vi "Test ReInit Negative Responce and ReInit.vi"(7 "Sequence Context In":refnum<k7>, 8 "error in":errorcluster, 9 "Test Mode":u16, 10 "LV PPS Config":T1={"VISA Resource"="", "Voltage Level (0.0 V)"=12.0, "CURRent Limit (0.0 A)"=6.0, "OVP LEVEL (0V)"=15.0, "Enable OVP (T: Enable)"=FALSE, "OCP LEVEL (0A)"=8.0, "Enable OCP (T: Enable)"=TRUE, "Value Out"="", "Value In"="", "Actual Voltage Level (V)"=-0.11, "Actual Current Limit (A)"=0.0, "Select Instrument"="", "Enable Output"=TRUE, "PPS Operation"=enum."Configure", "Type"=0} {"Type" items=["Voltage", "Current"]; "Actual Current Limit (A)" format="%.2f"; "Actual Voltage Level (V)" format="%.2f"; "OCP LEVEL (0A)" format="%.2f"; "OVP LEVEL (0V)" format="%.2f"; "Voltage Level (0.0 V)" format="%.2f"}, 11 "HV PPS Config":T1={"VISA Resource"="", "Voltage Level (0.0 V)"=48.0, "CURRent Limit (0.0 A)"=150.0, "OVP LEVEL (0V)"=55.0, "Enable OVP (T: Enable)"=FALSE, "OCP LEVEL (0A)"=160.0, "Enable OCP (T: Enable)"=TRUE, "Value Out"="", "Value In"="", "Actual Voltage Level (V)"=-0.11, "Actual Current Limit (A)"=0.0, "Select Instrument"="", "Enable Output"=TRUE, "PPS Operation"=enum."Configure", "Type"=0} {"Type" items=["Voltage", "Current"]; "Actual Current Limit (A)" format="%.2f"; "Actual Voltage Level (V)" format="%.2f"; "OCP LEVEL (0A)" format="%.2f"; "OVP LEVEL (0V)" format="%.2f"; "Voltage Level (0.0 V)" format="%.2f"}) -> (0 "error out":errorcluster, 2 "Response Code":u8[](array[numeric]), 3 "Positive Responce":bool)   [LabVIEW 2023, in "HardwareAbstractionLayer_LVOOP.lvlib" / "Wait Monitor.lvclass"]
uses:
  Wait Monitor.lvclass
  PowerSupply/Teststand/Control/PPS StepType Control.ctl
  Teststand Steptypes/CAN/STP/Steptypes/Control/STP Data.ctl
  CAN/CAN Application Protocols/STP Protocol_class/Ctrls/STP CMD.ctl
  Teststand Steptypes/DAQ/Relay Output/Control/Relay Output.ctl
  c292acb4-9eb8-428b-88b9-75ff1cad1871.vi
  57b82cc3-dd7c-4d3a-8ba9-81b38abffcad.vi
  725d82db-e125-4af1-8c31-2eddca650097.vi
  e56fdc52-0104-40be-a5d4-315e7d7fad48.vi
  ae1cdcb4-d38d-44ac-ba66-047396e49866.vi
  74cc3969-7d3f-4b2d-8c71-1ae829f8c662.vi
  02209c7f-5af8-4368-83f9-8143192c00df.vi
  Teststand/Teststand.lvclass
  CAN/CAN Application Protocols/STP Protocol_class/STP Protocol.lvclass
  Teststand Steptypes/LTT_TeststandSteptypes.lvlib
  PowerSupply/PowerSupply.lvclass
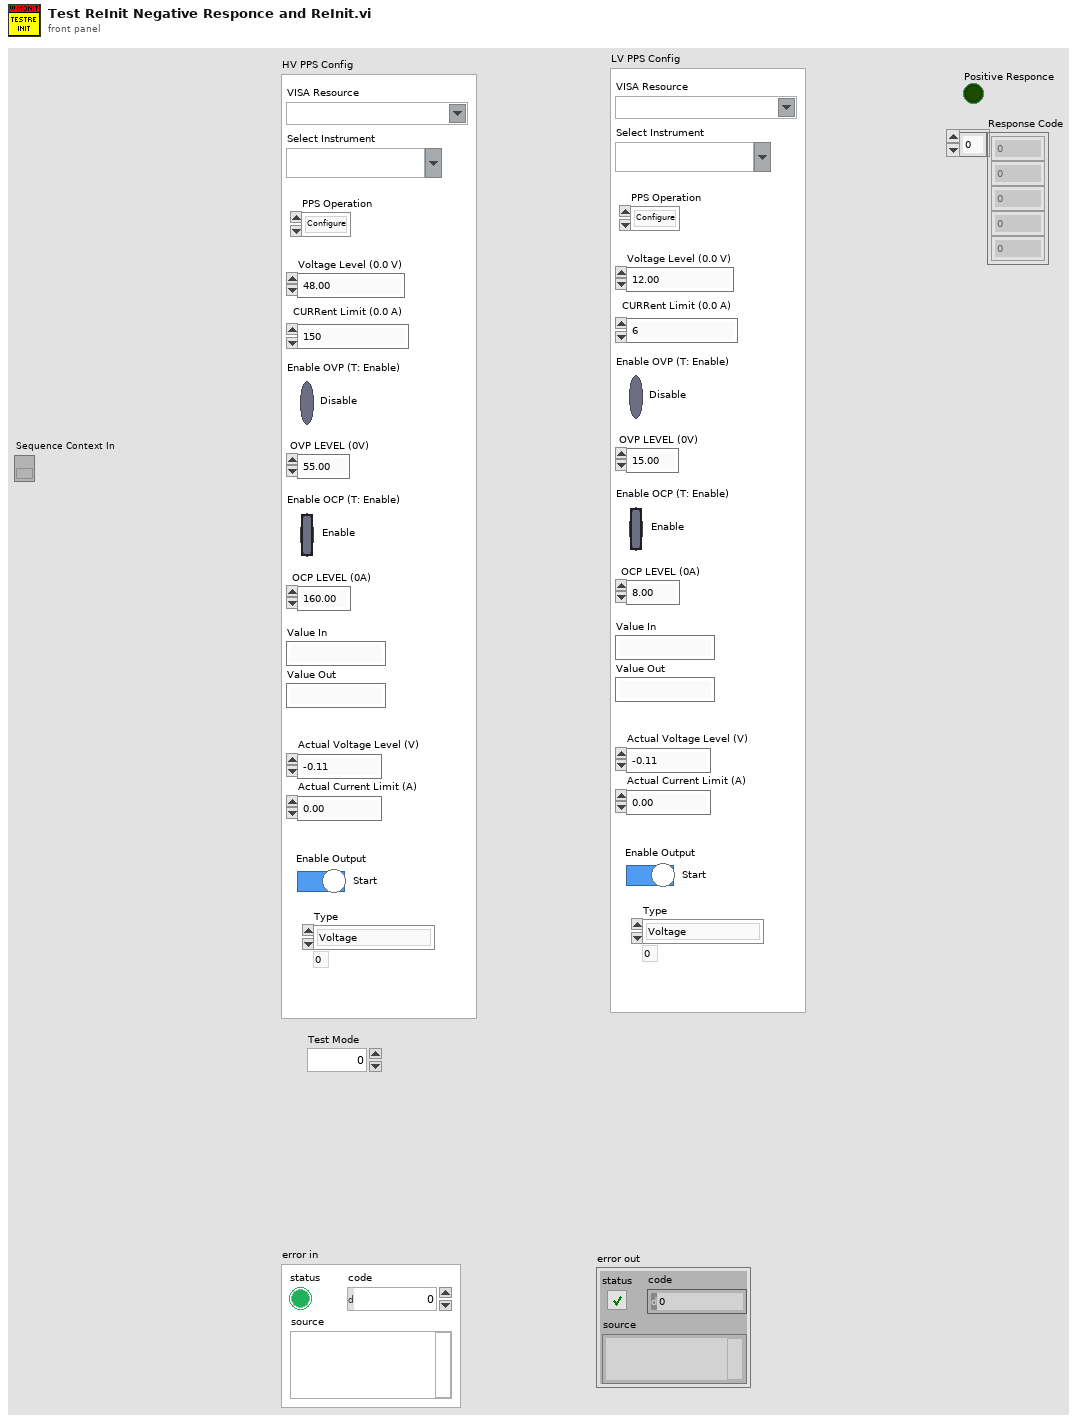
[diagram p1: front panel]
types:
  T1 = typedef "HardwareAbstractionLayer_LVOOP.lvlib/PowerSupply.lvclass/PPS StepType Control.ctl" = cluster{"VISA Resource":refnum<visa-resource-name>, "Voltage Level (0.0 V)":dbl, "CURRent Limit (0.0 A)":dbl, "OVP LEVEL (0V)":dbl, "Enable OVP (T: Enable)":bool, "OCP LEVEL (0A)":dbl, "Enable OCP (T: Enable)":bool, "Value Out":string, "Value In":string, "Actual Voltage Level (V)":dbl, "Actual Current Limit (A)":dbl, "Select Instrument":string, "Enable Output":bool, "PPS Operation":enum32{"Init", "Self Test", "Configure", "Measure", "Close"}, "Type":u16}
  T2 = enum32{"Init", "Self Test", "Configure", "Measure", "Close"}
  T3 = typedef "LTT_TeststandSteptypes.lvlib/STP Data.ctl" = cluster{"ECU CAN Port":string, "CMD":T4, "CAN Write Data":u8[], "Response Decoder":enum16{"String", "Number", "Boolean"}, "String":cluster{"Start Index":i32, "Length":i32}, "Number":cluster{"MSB Index":i32, "LSB Index":i32}, "Boolean":cluster{"Index":i32, "Bool":cluster{"7":bool, "6":bool, "5":bool, "4":bool, "3":bool, "2":bool, "1":bool, "0":bool, "7 Enabled":bool, "6 Enabled":bool, "5 Enabled":bool, "4 Enabled":bool, "3 Enabled":bool, "2 Enabled":bool, "1 Enabled":bool, "0 Enabled":bool}}}
  T4 = typedef "HardwareAbstractionLayer_LVOOP.lvlib/CAN Application Protocols Lib.lvlib/STP Protocol.lvclass/STP CMD.ctl" = u8
  T5 = typedef "LTT_TeststandSteptypes.lvlib/Relay Output.ctl" = cluster{"Signal Name List":cluster{"Signal Name":string, "Enable Output":bool}[]}
  T6 = typedef "HardwareAbstractionLayer_LVOOP.lvlib/Teststand.lvclass/Teststand Status Control.ctl" = cluster{"Terminating or Aborting":bool, "Stop":bool, "Socket Count":i16, "Selected Sockets":i16[]}
  T7 = typedef "LTT_TeststandSteptypes.lvlib/STP Out Data.ctl" = cluster{"String Data":string, "Numeric Data":dbl, "Boolean Data":bool, "RequestTimeout?":bool, "ResponseData":u8[], "PositiveResponse?":bool}
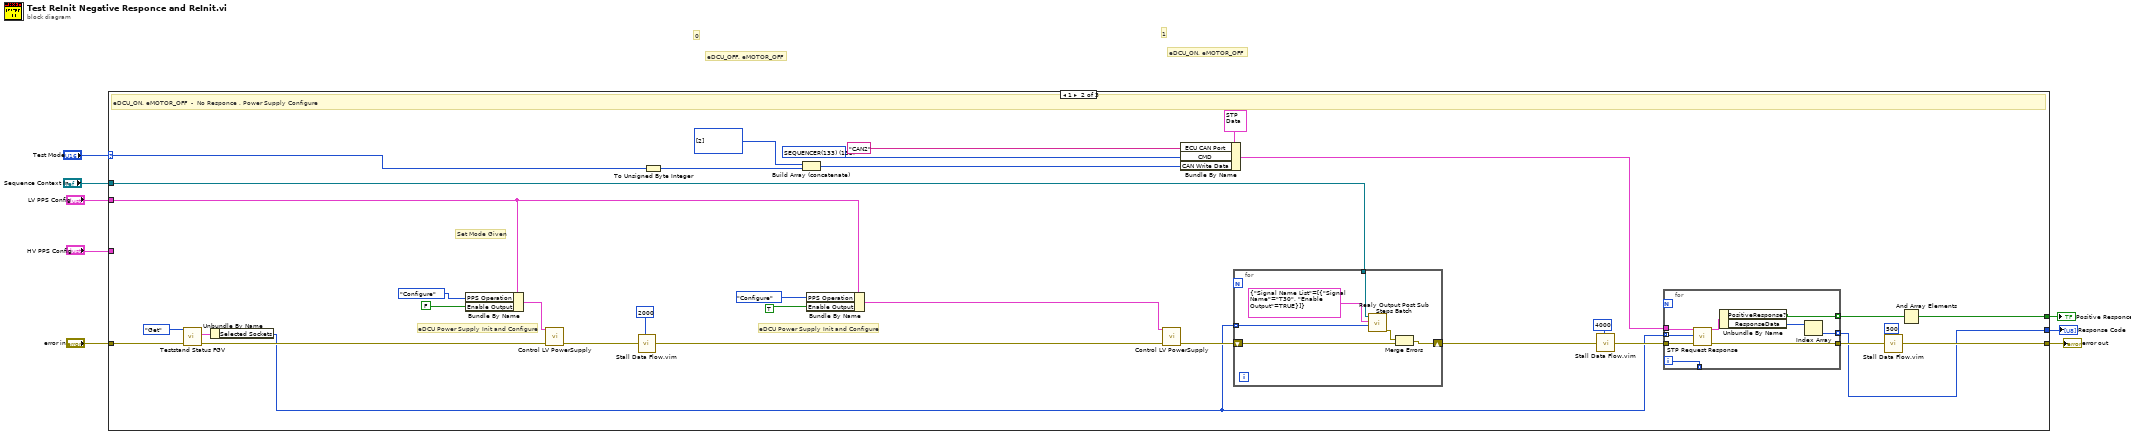
[diagram p0: block diagram]
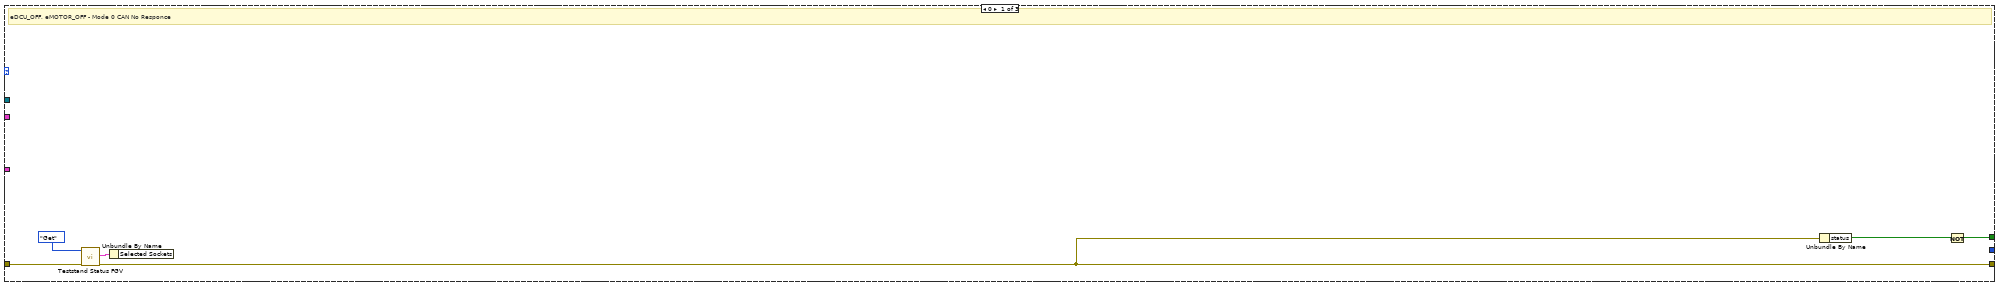
[diagram p2: hidden frame]
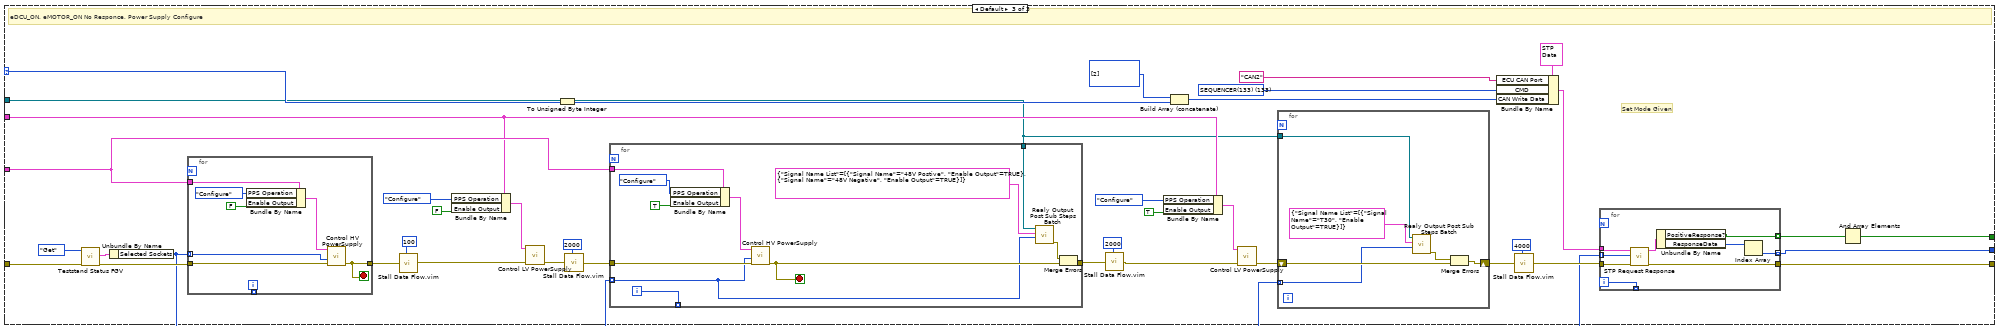
[diagram p3: hidden frame]
diagram:
  # "0"
  # "1"
  # "eDCU_ON, eMOTOR_OFF"
  # "eDCU_OFF, eMOTOR_OFF"
  n1 = case shown="1" "Test Mode" {
    selector: "Test Mode" -> [_ w36 w88]
    tunnel: "error in" -> [w12 w47 w99]
    tunnel: [w9 w32 w94] -> w7
    tunnel: "HV PPS Config" -> [_ _ w78]
    tunnel: "LV PPS Config" -> [_ w21 w70]
    tunnel: [w11 w30 w84] -> w3
    tunnel: [_ w29 w83] -> w2
    tunnel: "Sequence Context In" -> [_ w18 w64]
    frame 0 {
      # "eDCU_OFF, eMOTOR_OFF - Mode 0 CAN No Responce"
      n2 = call "Teststand Status FGV.vi"("error in"=w12, "Option"=enum16{"Set", "Get"}."Get") -> ("error out"=w9:errorcluster, "Teststand Status Out"=w13:T6)  [unwired: 8 in]
      n3 = Unbundle By Name(w13) -> ()  [unwired: 1 out]
      n4 = Unbundle By Name(w9) -> ("status"=w10:bool)
      n5 = Not(x=w10) -> (.not. x?=w11:bool)
    }
    frame 1 {
      w38 = T4 133 items=["TSW_VERSION(130)"=130, "WAIT_EVENT(132)"=132, "SEQUENCER(133)"=133, "TSW_RESET(150)"=150, "CONFIG_ECU(151)"=151, "TEST_CORE (152)"=152, "TEST_WATCHDOG (153)"=153, "TEST_MONITORING (154)"=154, "READ_MEMORY (162)"=162, "WRITE_ERASE_MEMORY (164)"=164, "COMM_EXTERNAL (190)"=190, "COMM_INTERNAL (195)"=195, "GET_ANALOG_INPUT (210)"=210, "GET_DIGITAL_INPUT (211)"=211, "GET_FREQUENCY_INPUT (212)"=212, "TEST_INPUT_STRUCTURE (214)"=214, "GENERATE_OUTPUT_SIGNAL (220)"=220, "GENERATE_SYNCHRONIZED_OUTPUT_SIGNALS (221)"=221, "eDCU_Specific (250)"=250] ("CMD")
      # "eDCU Power Supply Init and Configure"
      # "eDCU Power Supply Init and Configure"
      # "Set Mode Given"
      # "eDCU_ON, eMOTOR_OFF  -  No Responce , Power Supply Configure"
      n6 = call "Teststand Status FGV.vi"("error in"=w47, "Option"=enum16{"Set", "Get"}."Get") -> ("error out"=w46:errorcluster, "Teststand Status Out"=w48:T6)  [unwired: 8 in]
      n7 = Unbundle By Name(w48) -> ("Selected Sockets"=w15:i16[])
      n8 = Bundle By Name(cluster=w21, "PPS Operation"=T2."Configure", "Enable Output"=FALSE) -> (w28:T1)
      n9 = call "Control LV PowerSupply.vi"("error in"=w46, "PPS Config In"=w28) -> ("error out"=w27:errorcluster)  [unwired: 7 in, 2 out]
      n10 = call "Stall Data Flow.vim"("value in"=w27, "milliseconds to wait"=u32 2000) -> ("value out"=w20:errorcluster)  [unwired: 1 out]
      n11 = To Unsigned Byte Integer(number=w36) -> (unsigned 8bit integer=w35:u8)
      n12 = Build Array (concatenate)(u8[] [2] ("CAN Write Data"), w35) -> (w34:u8[])
      n13 = Bundle By Name(cluster=w21, "PPS Operation"=T2."Configure", "Enable Output"=TRUE) -> (w24:T1)
      n14 = call "Control LV PowerSupply.vi"("error in"=w20, "PPS Config In"=w24) -> ("error out"=w17:errorcluster)  [unwired: 7 in, 2 out]
      n15 = Bundle By Name(cluster=T3 {"ECU CAN Port"="CAN2", "CMD"=130, "CAN Write Data"=[], "Response Decoder"=enum."String", "String"={"Start Index"=0, "Length"=-1}, "Number"={"MSB Index"=0, "LSB Index"=1}, "Boolean"={"Index"=0, "Bool"={"7"=FALSE, "6"=FALSE, "5"=FALSE, "4"=FALSE, "3"=FALSE, "2"=FALSE, "1"=FALSE, "0"=FALSE, "7 Enabled"=FALSE, "6 Enabled"=FALSE, "5 Enabled"=FALSE, "4 Enabled"=FALSE, "3 Enabled"=FALSE, "2 Enabled"=FALSE, "1 Enabled"=FALSE, "0 Enabled"=FALSE}}} ("STP Data in"), "ECU CAN Port"="CAN2", "CMD"=w38, "CAN Write Data"=w34) -> (w40:T3)
      n16 = for {
        tunnel: w18 -> [w53]
        shift-right: [w51] -> w16
        shift-left: w17 -> [w52]
        tunnel: w15 -> [w49] mode=indexing
        n17 = call "Realy Output Post Sub Steps Batch.vi"("Socket No"=w49, "RelayOutputWrite"=T5 {"Signal Name List"=[{"Signal Name"="T30", "Enable Output"=TRUE}]}, "Sequence Context In"=w53) -> ("error out"=w50:errorcluster)  [unwired: 6 in, 2 out]
        n18 = Merge Errors(w50, w52) -> (w51:errorcluster)
      }
      n19 = call "Stall Data Flow.vim"("value in"=w16, "milliseconds to wait"=u32 4000) -> ("value out"=w42:errorcluster)  [unwired: 1 out]
      n20 = for {
        tunnel: w40 -> [w61]
        tunnel: [w60] -> _ mode=indexing
        tunnel: w15 -> [w59] mode=indexing
        tunnel: w42 -> [w62]
        tunnel: [w63] -> w43
        tunnel: [w57] -> w33 mode=indexing
        tunnel: [w55] -> w29 mode=indexing
        i -> [w60]
        n21 = call "STP Request Response.vi"("error in"=w62, "Socket No"=w59, "STP Data in"=w61) -> ("error out"=w63:errorcluster, "STP Data Out"=w58:T7)  [unwired: 5 in, 2 out]
        n22 = Unbundle By Name(w58) -> ("PositiveResponse?"=w57:bool, "ResponseData"=w56:u8[])
        n23 = Index Array(array=w56) -> (element=w55:u8)  [unwired: 1 in]
      }
      n24 = call "Stall Data Flow.vim"("value in"=w43, "milliseconds to wait"=u32 500) -> ("value out"=w32:errorcluster)  [unwired: 1 out]
      n25 = And Array Elements(Boolean array=w33) -> (logical AND=w30:bool)
    }
    frame Default {
      w90 = T4 133 items=["TSW_VERSION(130)"=130, "WAIT_EVENT(132)"=132, "SEQUENCER(133)"=133, "TSW_RESET(150)"=150, "CONFIG_ECU(151)"=151, "TEST_CORE (152)"=152, "TEST_WATCHDOG (153)"=153, "TEST_MONITORING (154)"=154, "READ_MEMORY (162)"=162, "WRITE_ERASE_MEMORY (164)"=164, "COMM_EXTERNAL (190)"=190, "COMM_INTERNAL (195)"=195, "GET_ANALOG_INPUT (210)"=210, "GET_DIGITAL_INPUT (211)"=211, "GET_FREQUENCY_INPUT (212)"=212, "TEST_INPUT_STRUCTURE (214)"=214, "GENERATE_OUTPUT_SIGNAL (220)"=220, "GENERATE_SYNCHRONIZED_OUTPUT_SIGNALS (221)"=221, "eDCU_Specific (250)"=250] ("CMD")
      # "Set Mode Given"
      # "eDCU_ON, eMOTOR_ON No Responce, Power Supply Configure"
      n26 = call "Teststand Status FGV.vi"("error in"=w99, "Option"=enum16{"Set", "Get"}."Get") -> ("error out"=w100:errorcluster, "Teststand Status Out"=w101:T6)  [unwired: 8 in]
      n27 = Unbundle By Name(w101) -> ("Selected Sockets"=w65:i16[])
      n28 = for {
        tunnel: w100 -> [w132]
        tunnel: [w137] -> w98
        tunnel: w65 -> [w136] mode=indexing
        tunnel: w78 -> [w135]
        tunnel: [w131] -> _ mode=indexing
        i -> [w131]
        stop <- w137 stop-if-true
        n29 = Bundle By Name(cluster=w135, "PPS Operation"=T2."Configure", "Enable Output"=FALSE) -> (w134:T1)
        n30 = call "Control HV PowerSupply.vi"("error in"=w132, "Socket Index"=w136, "PPS Config In"=w134) -> ("error out"=w137:errorcluster)  [unwired: 6 in, 2 out]
      }
      n31 = call "Stall Data Flow.vim"("value in"=w98, "milliseconds to wait"=u32 100) -> ("value out"=w82:errorcluster)  [unwired: 1 out]
      n32 = Bundle By Name(cluster=w70, "PPS Operation"=T2."Configure", "Enable Output"=FALSE) -> (w81:T1)
      n33 = call "Control LV PowerSupply.vi"("error in"=w82, "PPS Config In"=w81) -> ("error out"=w80:errorcluster)  [unwired: 7 in, 2 out]
      n34 = To Unsigned Byte Integer(number=w88) -> (unsigned 8bit integer=w87:u8)
      n35 = call "Stall Data Flow.vim"("value in"=w80, "milliseconds to wait"=u32 2000) -> ("value out"=w77:errorcluster)  [unwired: 1 out]
      n36 = for {
        tunnel: w77 -> [w116]
        tunnel: [w110] -> w75
        tunnel: w65 -> [w111] mode=indexing
        tunnel: w78 -> [w119]
        tunnel: [w115] -> _ mode=indexing
        tunnel: w64 -> [w112]
        i -> [w115]
        stop <- w120 stop-if-true
        n37 = Bundle By Name(cluster=w119, "PPS Operation"=T2."Configure", "Enable Output"=TRUE) -> (w118:T1)
        n38 = call "Control HV PowerSupply.vi"("error in"=w116, "Socket Index"=w111, "PPS Config In"=w118) -> ("error out"=w120:errorcluster)  [unwired: 6 in, 2 out]
        n39 = call "Realy Output Post Sub Steps Batch.vi"("Socket No"=w111, "RelayOutputWrite"=T5 {"Signal Name List"=[{"Signal Name"="48V Postive", "Enable Output"=TRUE}, {"Signal Name"="48V Negative", "Enable Output"=TRUE}]}, "Sequence Context In"=w112) -> ("error out"=w109:errorcluster)  [unwired: 6 in, 2 out]
        n40 = Merge Errors(w109, w120) -> (w110:errorcluster)
      }
      n41 = call "Stall Data Flow.vim"("value in"=w75, "milliseconds to wait"=u32 2000) -> ("value out"=w71:errorcluster)  [unwired: 1 out]
      n42 = Bundle By Name(cluster=w70, "PPS Operation"=T2."Configure", "Enable Output"=TRUE) -> (w73:T1)
      n43 = Build Array (concatenate)(u8[] [2] ("CAN Write Data"), w87) -> (w86:u8[])
      n44 = call "Control LV PowerSupply.vi"("error in"=w71, "PPS Config In"=w73) -> ("error out"=w67:errorcluster)  [unwired: 7 in, 2 out]
      n45 = for {
        shift-right: [w104] -> w66
        shift-left: w67 -> [w108]
        tunnel: w65 -> [w105] mode=indexing
        tunnel: w64 -> [w106]
        n46 = call "Realy Output Post Sub Steps Batch.vi"("Socket No"=w105, "RelayOutputWrite"=T5 {"Signal Name List"=[{"Signal Name"="T30", "Enable Output"=TRUE}]}, "Sequence Context In"=w106) -> ("error out"=w103:errorcluster)  [unwired: 6 in, 2 out]
        n47 = Merge Errors(w103, w108) -> (w104:errorcluster)
      }
      n48 = Bundle By Name(cluster=T3 {"ECU CAN Port"="CAN2", "CMD"=130, "CAN Write Data"=[], "Response Decoder"=enum."String", "String"={"Start Index"=0, "Length"=-1}, "Number"={"MSB Index"=0, "LSB Index"=1}, "Boolean"={"Index"=0, "Bool"={"7"=FALSE, "6"=FALSE, "5"=FALSE, "4"=FALSE, "3"=FALSE, "2"=FALSE, "1"=FALSE, "0"=FALSE, "7 Enabled"=FALSE, "6 Enabled"=FALSE, "5 Enabled"=FALSE, "4 Enabled"=FALSE, "3 Enabled"=FALSE, "2 Enabled"=FALSE, "1 Enabled"=FALSE, "0 Enabled"=FALSE}}} ("STP Data in"), "ECU CAN Port"="CAN2", "CMD"=w90, "CAN Write Data"=w86) -> (w92:T3)
      n49 = call "Stall Data Flow.vim"("value in"=w66, "milliseconds to wait"=u32 4000) -> ("value out"=w68:errorcluster)  [unwired: 1 out]
      n50 = for {
        tunnel: w92 -> [w127]
        tunnel: [w126] -> _ mode=indexing
        tunnel: w65 -> [w125] mode=indexing
        tunnel: w68 -> [w128]
        tunnel: [w129] -> w94
        tunnel: [w123] -> w85 mode=indexing
        tunnel: [w121] -> w83 mode=indexing
        i -> [w126]
        n51 = call "STP Request Response.vi"("error in"=w128, "Socket No"=w125, "STP Data in"=w127) -> ("error out"=w129:errorcluster, "STP Data Out"=w124:T7)  [unwired: 5 in, 2 out]
        n52 = Unbundle By Name(w124) -> ("PositiveResponse?"=w123:bool, "ResponseData"=w122:u8[])
        n53 = Index Array(array=w122) -> (element=w121:u8)  [unwired: 1 in]
      }
      n54 = And Array Elements(Boolean array=w85) -> (logical AND=w84:bool)
    }
  }
  "error out" <- w7
  "Positive Responce" <- w3
  "Response Code" <- w2
